vi "2.1 Helper - Generate RegEx.vi"(1 "# Datums":i32) -> (0 "RegEx":string)   [LabVIEW 2011]
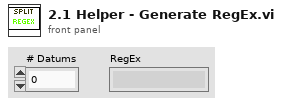
[diagram p1: front panel]
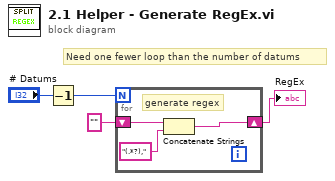
[diagram p0: block diagram]
diagram:
  # "Need one fewer loop than the number of datums"
  n1 = Decrement(x="# Datums") -> (x-1=w1:i32)
  n2 = for {
    N: w1 -> [_]
    shift-right: [w5] -> w4
    shift-left: "" -> [w7]
    # "generate regex"
    n3 = Concatenate Strings(w7, "(.*?),") -> (w5:string)
  }
  "RegEx" <- w4
